vi "Read backgroundColor.vi"(8 "error in (no error)":errorcluster, 11 "TextDecoration in":refnum<class "TextDecoration.lvclass">) -> (0 "error out":errorcluster, 2 "backgroundColor":u32(colorbox), 3 "TextDecoration out":refnum<class "TextDecoration.lvclass">)   [LabVIEW 2023, in "TLC_Scripto.lvlib" / "TextDecoration.lvclass"]
uses:
  TextDecoration.lvclass
  TextDecoration.lvclass/TextDecoration.ctl
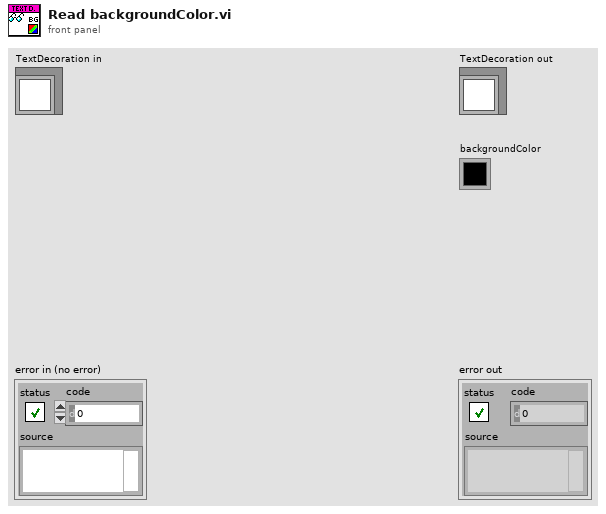
[diagram p1: front panel]
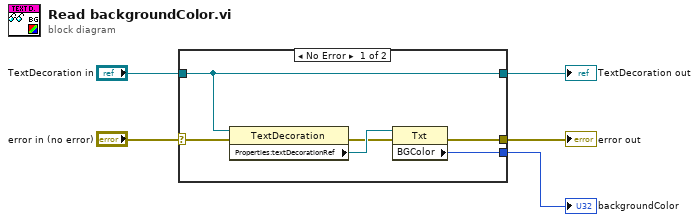
[diagram p0: block diagram]
diagram:
  n1 = case shown="No Error" "error in (no error)" {
    selector: "error in (no error)" -> [w7 w12]
    tunnel: [w6 w12] -> w4
    tunnel: [w11 w13] -> w2
    tunnel: "TextDecoration in" -> [w11 w13]
    tunnel: [w9 _] -> w1
    frame No Error {
      n2 = property class="TextDecoration"(reference=w11, error in=w7) -> (error out=w8:errorcluster, "Properties:textDecorationRef"=w10:refnum<vi>)  [unwired: 1 out]
      n3 = property class="Txt"(reference=w10, error in=w8) -> (error out=w6:errorcluster, "BGColor"=w9:u32)  [unwired: 1 out]
    }
    frame Error {
    }
  }
  "error out" <- w4
  "TextDecoration out" <- w2
  "backgroundColor" <- w1
